vi "ISM Reserve Pump.vi"(8 "error in (no error)":errorcluster, 10 "ISM Channel # In":i32, 11 "ISM Pump # In":i32) -> (0 "error out":errorcluster, 3 "ISM Pump # Out":i32)   [LabVIEW 2018, in "Ismatec 4308.lvlib"]
uses:
  Ismatec 4308.lvlib
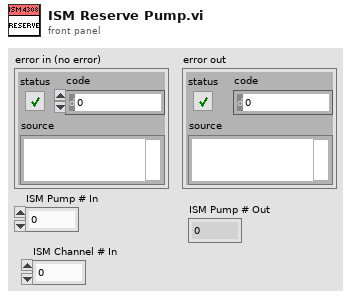
[diagram p1: front panel]
types:
  T1 = cluster{"Busy":bool, "ChannelCnt":dbl, "Initialized":bool, "Current Channel":dbl, "Initialized Channels":dbl[]}[]
  T2 = cluster{"Busy":bool, "ChannelCnt":dbl, "Initialized":bool, "Current Channel":dbl, "Initialized Channels":dbl[]}
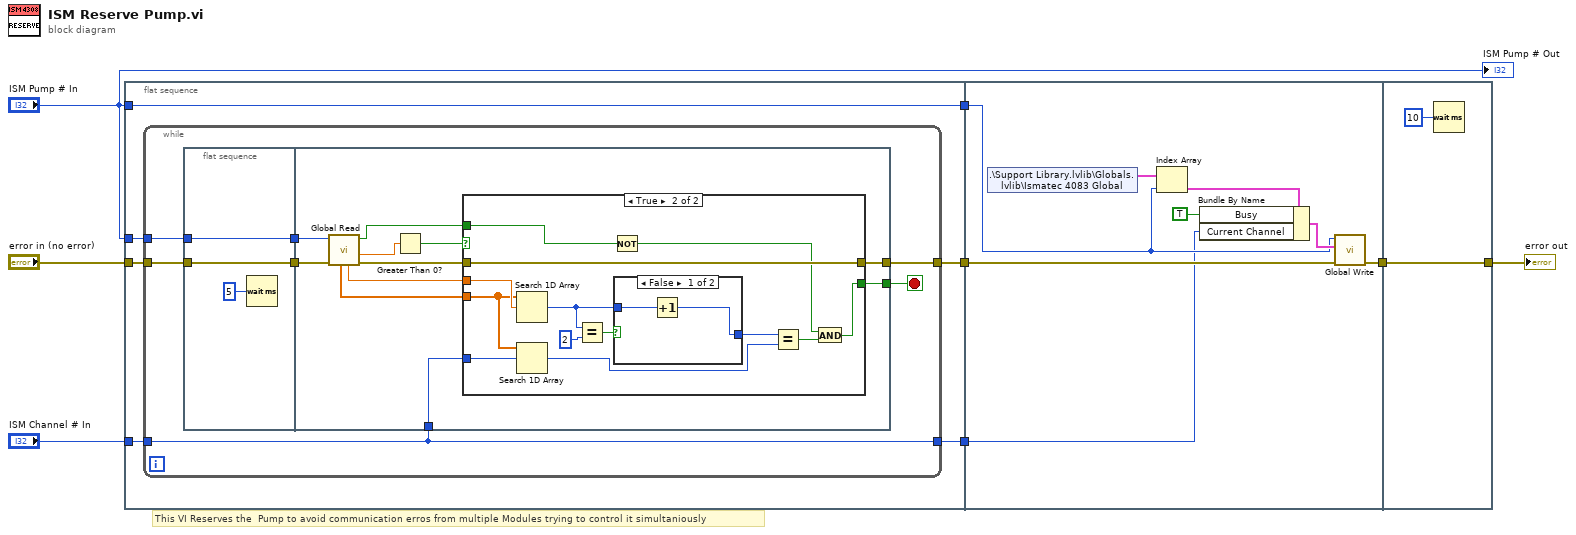
[diagram p0: block diagram]
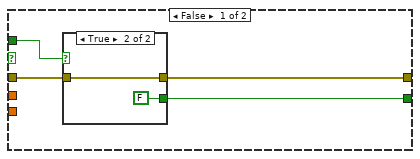
[diagram p2: hidden frame]
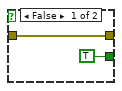
[diagram p3: hidden frame]
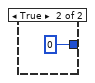
[diagram p4: hidden frame]
diagram:
  # "This VI Reserves the  Pump to avoid communication erros from multiple Modules trying to control it simultaniously"
  n1 = flat-sequence {
    tunnel: "ISM Pump # In" -> [w14]
    tunnel: [w11] -> w6
    tunnel: [w14] -> w5
    tunnel: "ISM Pump # In" -> [w13]
    tunnel: "error in (no error)" -> [w12]
    tunnel: "ISM Channel # In" -> [w10]
    tunnel: [w9] -> w1
    tunnel: [w66] -> w8
    tunnel: w6 -> [w67]
    tunnel: w5 -> [w61]
    tunnel: w1 -> [w60]
    tunnel: [w69] -> w7
    tunnel: w8 -> [w69]
    frame #0 {
      n2 = while {
        tunnel: w13 -> [w17]
        tunnel: [w21] -> w11
        tunnel: w12 -> [w18]
        tunnel: w10 -> [w15]
        tunnel: [w15] -> w9
        stop <- w20 stop-if-true
        n3 = flat-sequence {
          tunnel: [w24] -> w19
          tunnel: w18 -> [w24]
          tunnel: w17 -> [w23]
          tunnel: [w23] -> w16
          tunnel: [w28] -> w21
          tunnel: [w30] -> w20
          tunnel: w19 -> [w35]
          tunnel: w16 -> [w34]
          tunnel: w15 -> [w27]
          frame #0 {
            n4 = Wait (ms)(milliseconds to wait=u32 5) -> ()  [unwired: 1 out]
          }
          frame #1 {
            n5 = call "Global Read.vi"("error in (no error)"=w35, "Pump Number"=w34) -> ("error out"=w29:errorcluster, "ChannelCnt"=w32:dbl, "Busy"=w31:bool, "Current Channel"=w26:dbl, "Initialized Channels"=w25:dbl[])  [unwired: 3 in, 2 out]
            n6 = Greater Than 0?(x=w32) -> (x > 0?=w33:bool)
            n7 = case shown="True" w33 {
              tunnel: w31 -> [w39 w50]
              tunnel: [w38 w49] -> w30
              tunnel: w29 -> [w37 w51]
              tunnel: [w36 w51] -> w28
              tunnel: w25 -> [_ w54]
              tunnel: w27 -> [_ w56]
              tunnel: w26 -> [_ w55]
              frame False {
                n8 = case shown="True" w39 {
                  tunnel: [TRUE FALSE] -> w38
                  tunnel: w37 -> [w40 w42]
                  tunnel: [w40 w42] -> w36
                  frame False {
                  }
                  frame True {
                  }
                }
              }
              frame True {
                n9 = Search 1D Array(1D array=w54, element=w55) -> (index of element=w48:i32)  [unwired: 1 in]
                n10 = Search 1D Array(1D array=w54, element=w56) -> (index of element=w52:i32)  [unwired: 1 in]
                n11 = Equal?(x=w48, y=2) -> (x = y?=w46:bool)
                n12 = Not(x=w50) -> (.not. x?=w44:bool)
                n13 = case shown="False" w46 {
                  tunnel: [w58 0] -> w53
                  tunnel: w48 -> [w57 _]
                  frame False {
                    n14 = Increment(x=w57) -> (x+1=w58:i32)
                  }
                  frame True {
                  }
                }
                n15 = Equal?(x=w53, y=w52) -> (x = y?=w45:bool)
                n16 = And(x=w44, y=w45) -> (x .and. y?=w49:bool)
              }
            }
          }
        }
      }
    }
    frame #1 {
      n17 = shared-variable ".\\Support Library.lvlib\\Globals.lvlib\\Ismatec 4083 Global"() -> (w65:T1)  [unwired: 1 in, 1 out]
      n18 = Index Array(array=w65, index=w61) -> (element=w62:T2)
      n19 = Bundle By Name(cluster=w62, "Busy"=TRUE, "Current Channel"=w60) -> (w63:T2)
      n20 = call "Global Write.vi"("error in (no error)"=w67, "Incoming Cluster"=w63, "Pump Number In"=w61) -> ("error out"=w66:errorcluster)  [unwired: 7 in, 1 out]
    }
    frame #2 {
      n21 = Wait (ms)(milliseconds to wait=u32 10) -> ()  [unwired: 1 out]
    }
  }
  "error out" <- w7
  "ISM Pump # Out" <- "ISM Pump # In"
